vi "Distribute 5-bar Torque.vi"(8 "error in (no error)":errorcluster, 10 "joint_torques":dbl[](array[numeric]), 11 "Finger in":refnum<class "Finger.lvclass">) -> (0 "error out":errorcluster, 2 "motor_torques":dbl[](array[numeric]), 3 "Finger out":refnum<class "Finger.lvclass">)   [LabVIEW 2011, in "Finger.lvclass"]
uses:
  Finger.lvclass
  Finger.lvclass/Finger.ctl
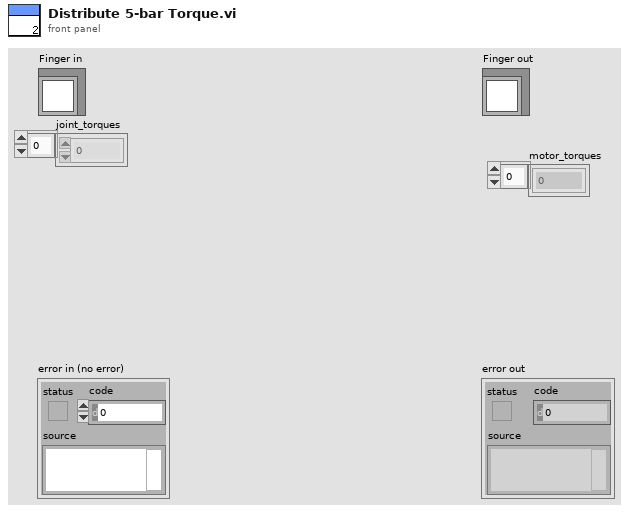
[diagram p1: front panel]
types:
  T1 = cluster{"L1":dbl, "L2":dbl, "L3":dbl, "L4":dbl, "d":dbl}
  T2 = cluster{"phi":dbl, "theta":dbl, "psi":dbl, "alpha":dbl}
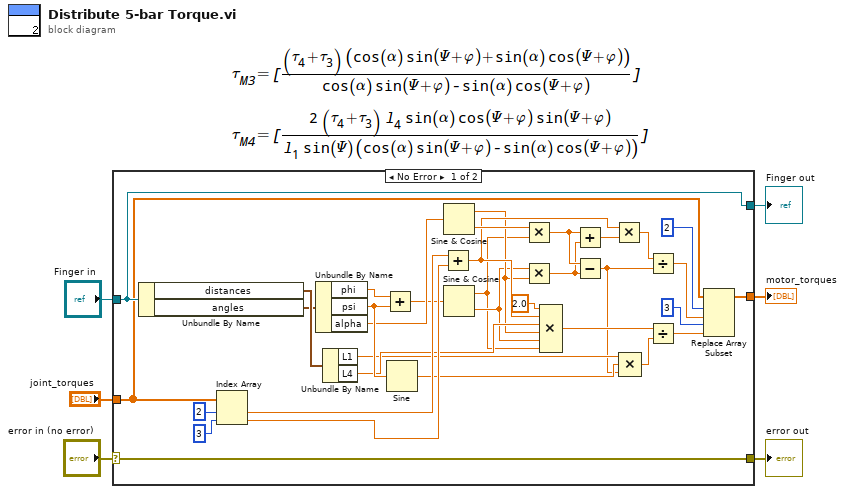
[diagram p0: block diagram]
diagram:
  n1 = case shown="No Error" "error in (no error)" {
    selector: "error in (no error)" -> [w40 w42]
    tunnel: [w40 w42] -> w5
    tunnel: [w39 w41] -> w3
    tunnel: "Finger in" -> [w39 w41]
    tunnel: [w27 _] -> w1
    tunnel: "joint_torques" -> [w28 _]
    frame No Error {
      n2 = Unbundle By Name(w39) -> ("distances"=w38:T1, "angles"=w37:T2)
      n3 = Index Array(array=w28, index #1=2 ("index"), index #2=3 ("index")) -> (element #1=w34:dbl, element #2=w33:dbl)
      n4 = Unbundle By Name(w37) -> ("phi"=w32:dbl, "psi"=w31:dbl, "alpha"=w30:dbl)
      n5 = Unbundle By Name(w38) -> ("L1"=w10:dbl, "L4"=w16:dbl)
      n6 = Add(x=w32, y=w31) -> (x+y=w29:dbl)
      n7 = Sine(x=w31) -> (sin(x)=w9:dbl)
      n8 = Add(x=w34, y=w33) -> (x+y=w18:dbl)
      n9 = Sine & Cosine(0:w30) -> (1:w15:dbl, 2:w24:dbl)
      n10 = Sine & Cosine(0:w29) -> (1:w13:dbl, 2:w14:dbl)
      n11 = Multiply(x=w24, y=w13) -> (x*y=w21:dbl)
      n12 = Multiply(x=w14, y=w15) -> (x*y=w20:dbl)
      n13 = Compound Arithmetic op=MULTIPLY(2.0 ("value"), w18, w16, w15, w14, w13) -> (w12:dbl)
      n14 = Add(x=w21, y=w20) -> (x+y=w23:dbl)
      n15 = Subtract(x=w21, y=w20) -> (x-y=w8:dbl)
      n16 = Multiply(x=w18, y=w23) -> (x*y=w22:dbl)
      n17 = Compound Arithmetic op=MULTIPLY(w10, w9, w8) -> (w7:dbl)
      n18 = Divide(x=w22, y=w8) -> (x/y=w19:dbl)
      n19 = Divide(x=w12, y=w7) -> (x/y=w11:dbl)
      n20 = Replace Array Subset(array=w28, new element #1=w19, index #1=2 ("index"), new element #2=w11, index #2=3 ("index")) -> (w27:dbl[])
    }
    frame Error {
    }
  }
  "error out" <- w5
  "Finger out" <- w3
  "motor_torques" <- w1
